vi "PPR_DRIVE_Wheel_ACT.vi"(6 "Pass_Through_Time":dbl=-1.0 format="%33.4f", 9 "Wheel Speed M/S":dbl, 10 "Wheel Speed Dmd M/S":dbl, 11 "Diff Wheel TypDef":T1) -> (3 "Wheel Motor Dmd":dbl, 4 "WheelSpeedErr":dbl, 7 "Limited Speed Dmd M/S":dbl)   [LabVIEW 2019]
uses:
  PPR_DRIVE_Wheel_TYPDEF.ctl
  <vilib>/Rock Robotics/WPI/MotorControl/WPI_MotorControlDeviceRef.ctl
  <vilib>/Rock Robotics/WPI/MotorControl/WPI_MotorControlType.ctl
  <vilib>/Rock Robotics/SystemInterfaces/DIO/FPGA_DIOPWMChannel.ctl
  <vilib>/Rock Robotics/WPI/PWM/WPI_PWMDeadband.ctl
  <vilib>/Rock Robotics/SystemInterfaces/DIO/FPGA_DIOChannel.ctl
  <vilib>/Rock Robotics/WPI/Encoder/WPI_EncoderDevRef.ctl
  <vilib>/Rock Robotics/SystemInterfaces/Encoder/FPGA_EncoderIdx.ctl
  <vilib>/Rock Robotics/SystemInterfaces/Counter/FPGA_CounterCtrSystemIndex.ctl
  <vilib>/Rock Robotics/WPI/Encoder/WPI_EncoderType.ctl
  <vilib>/Rock Robotics/WPI/ThirdParty/JAS_Junk/TrajLib/VI/Util_GetTime_U32.vi
  <vilib>/Rock Robotics/WPI/ThirdParty/JAS_Junk/TrajLib/SlewRateLimiter_New.vi
  <vilib>/Rock Robotics/WPI/ThirdParty/JAS_Junk/TrajLib/SlewRateLimiter_Reset.vi
  <vilib>/Rock Robotics/WPI/ThirdParty/JAS_Junk/TrajLib/SlewRateLimiter_Calculate.vi
  <vilib>/Rock Robotics/WPI/ThirdParty/JAS_Junk/TrajLib/SlewRateLimiter_SetRate.vi
  <vilib>/Rock Robotics/WPI/ThirdParty/JAS_Junk/TrajLib/SimpleMotorFF_Calculate.vi
  <vilib>/Rock Robotics/WPI/ThirdParty/JAS_Junk/TrajLib/PIDController_AtSetpoint.vi
  <vilib>/Rock Robotics/WPI/ThirdParty/JAS_Junk/TrajLib/PIDController_SetPIDF.vi
  <vilib>/Rock Robotics/WPI/ThirdParty/JAS_Junk/TrajLib/PIDController_SetDerivativeFilter.vi
  <vilib>/Rock Robotics/WPI/ThirdParty/JAS_Junk/TrajLib/PIDController_SetIntegratorRange.vi
  <vilib>/Rock Robotics/WPI/ThirdParty/JAS_Junk/TrajLib/PIDController_SetTolerancePandV.vi
  <vilib>/Rock Robotics/WPI/ThirdParty/JAS_Junk/TrajLib/PIDController_DisableContinousInput.vi
  <vilib>/Rock Robotics/WPI/ThirdParty/JAS_Junk/TrajLib/PIDController_EnableContinousInput.vi
  <vilib>/Rock Robotics/WPI/ThirdParty/JAS_Junk/TrajLib/PIDController_Reset.vi
  <vilib>/Rock Robotics/WPI/ThirdParty/JAS_Junk/TrajLib/PIDController_New.vi
  <vilib>/Rock Robotics/WPI/ThirdParty/JAS_Junk/TrajLib/PIDController_SetOutputLimits.vi
  <vilib>/Rock Robotics/WPI/ThirdParty/JAS_Junk/TrajLib/PIDController_NewPeriod.vi
  <vilib>/Rock Robotics/SystemInterfaces/NetworkCommunication/NetComm_UsageReport_report.vi
  <vilib>/Rock Robotics/WPI/ThirdParty/JAS_Junk/TrajLib/VI/Util_GetTime_U64.vi
  PPR_DRIVE_GLOBALS.vi
  <vilib>/Rock Robotics/WPI/ThirdParty/JAS_Junk/TrajLib/Globals/Util_LibraryGlobals.vi
  <vilib>/Rock Robotics/WPI/ThirdParty/JAS_Junk/TrajLib/PIDController_AdvCalculate_FF_Sp_Pv.vi
  <vilib>/Rock Robotics/WPI/ThirdParty/JAS_Junk/TrajLib/Trajectory_Library.lvlib
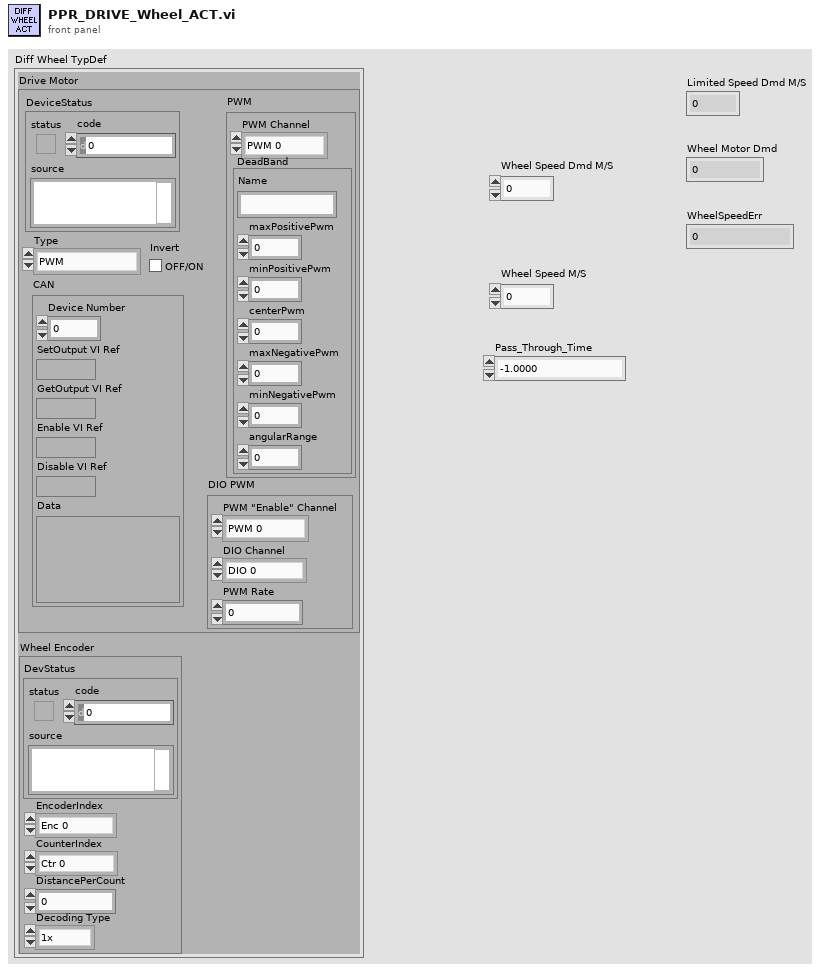
[diagram p1: front panel]
types:
  T1 = typedef "PPR_DRIVE_Wheel_TYPDEF.ctl" = cluster{"Drive Motor":T2, "Wheel Encoder":T7}
  T2 = typedef "WPI_MotorControlDeviceRef.ctl" = cluster{"DeviceStatus":errorcluster, "Type":T3, "PWM":cluster{"PWM Channel":T4, "DeadBand":T5}, "CAN":cluster{"Device Number":u8, "SetOutput VI Ref":variant, "GetOutput VI Ref":variant, "Enable VI Ref":variant, "Disable VI Ref":variant, "Data":variant}, "Invert":bool, "DIO PWM":cluster{"PWM \"Enable\" Channel":T4, "DIOChannel":T6, "PWM Rate":dbl}}
  T3 = typedef "WPI_MotorControlType.ctl" = enum16{"PWM", "CAN", "DIO PWM"}
  T4 = typedef "FPGA_DIOPWMChannel.ctl" = enum8{"PWM 0", "PWM 1", "PWM 2", "PWM 3", "PWM 4", "PWM 5", "PWM 6", "PWM 7", "PWM 8", "PWM 9", "PWM MXP 0", "PWM MXP 1", "PWM MXP 2", "PWM MXP 3", "PWM MXP 4", "PWM MXP 5", "PWM MXP 6", "PWM MXP 7", "PWM MXP 8", "PWM MXP 9", "Invalid"}
  T5 = typedef "WPI_PWMDeadband.ctl" = cluster{"Name":string, "maxPositivePwm":i32, "minPositivePwm":i32, "centerPwm":i32, "maxNegativePwm":i32, "minNegativePwm":i32, "angularRange":u16}
  T6 = typedef "FPGA_DIOChannel.ctl" = enum8{"DIO 0", "DIO 1", "DIO 2", "DIO 3", "DIO 4", "DIO 5", "DIO 6", "DIO 7", "DIO 8", "DIO 9", "DIO MXP 0", "DIO MXP 1", "DIO MXP 2", "DIO MXP 3", "DIO MXP 4", "DIO MXP 5", "DIO MXP 6", "DIO MXP 7", "DIO MXP 8", "DIO MXP 9", "DIO MXP 10", "DIO MXP 11", "DIO MXP 12", "DIO MXP 13", "DIO MXP 14", "DIO MXP 15", "SPI Port CS1", "SPI Port CS2", "SPI Port CS3", "SPI Port MISO", "SPI Port MOSI", "Invalid"}
  T7 = typedef "WPI_EncoderDevRef.ctl" = cluster{"DevStatus":errorcluster, "EncoderIndex":T8, "CounterIndex":T9, "DistancePerCount":dbl, "Decoding Type":T10}
  T8 = typedef "FPGA_EncoderIdx.ctl" = enum8{"Enc 0", "Enc 1", "Enc 2", "Enc 3", "Enc 4", "Enc 5", "Enc 6", "Enc 7", "Invalid"}
  T9 = typedef "FPGA_CounterCtrSystemIndex.ctl" = enum8{"Ctr 0", "Ctr 1", "Ctr 2", "Ctr 3", "Ctr 4", "Ctr 5", "Ctr 6", "Ctr 7", "Invalid"}
  T10 = typedef "WPI_EncoderType.ctl" = enum16{"1x", "2x", "4x"}
  T11 = typedef "Trajectory_Library.lvlib/SIMPLE_MOTOR_FF.ctl" = cluster{"Ks":dbl, "Kv":dbl, "Ka":dbl, "KnInv":dbl}
  T12 = typedef "Trajectory_Library.lvlib/PID_ADV_LIMITS.ctl" = cluster{"MaxInput":dbl, "MinInput":dbl, "Continuous":bool, "MaxOutput":dbl, "MinOutput":dbl}
  T13 = typedef "Trajectory_Library.lvlib/PID_ADV_TUNING.ctl" = cluster{"Kf":dbl, "Kp":dbl, "Ki":dbl, "Kd":dbl, "MaximumIntegral":dbl, "MinimumIntegral":dbl, "Filter Derivative":bool}
  T14 = typedef "Trajectory_Library.lvlib/PID_CONTROLLER.ctl" = cluster{"Kp":dbl, "Ki":dbl, "Kd":dbl, "Period":dbl, "Max_Integral":dbl, "Min_Integral":dbl, "Max_Input":dbl, "Min_Input":dbl, "Continuous":bool, "PositionError":dbl, "VelocityError":dbl, "PrevError":dbl, "TotalError":dbl, "PositionTolerance":dbl, "VelocityTolerance":dbl, "SetPoint":dbl, "Kf":dbl, "Prev_Deriv":dbl, "Prev_Deriv 2":dbl, "DerivativeFilter":bool, "Min_Output":dbl, "Max_Output":dbl, "Prev_F_P":dbl, "Prev_F_P_2":dbl, "AntiWindupActive":bool, "Measurement":dbl}
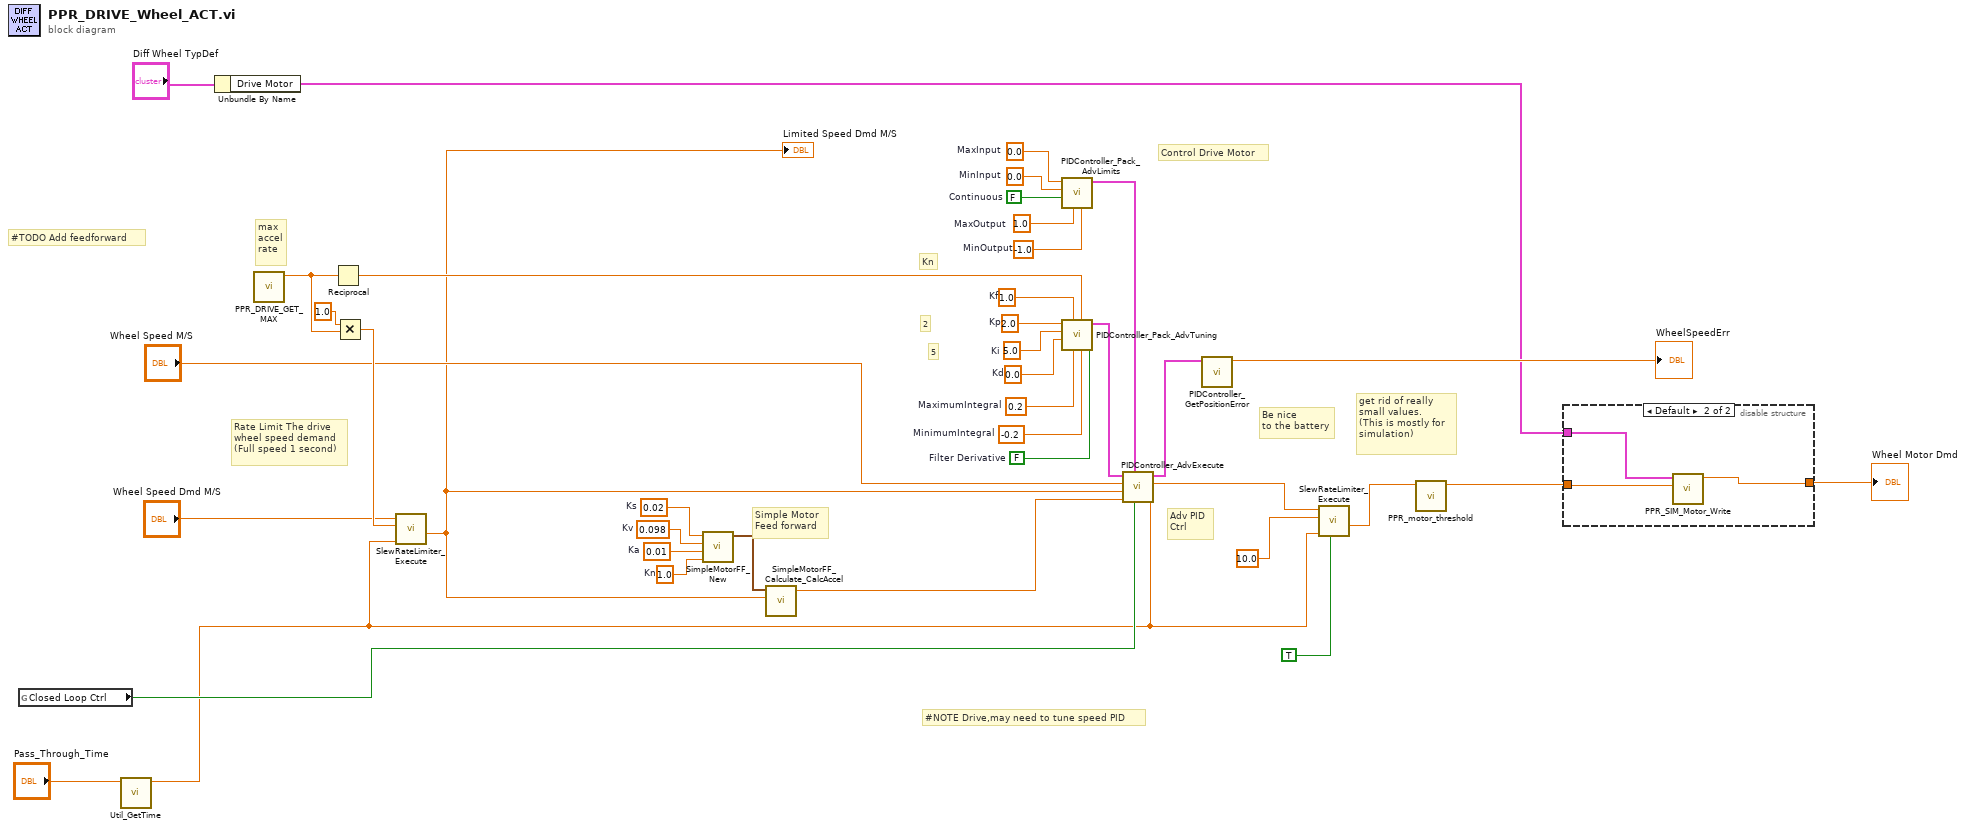
[diagram p0: block diagram]
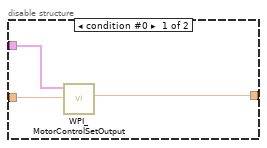
[diagram p2: hidden frame]
diagram:
  w7 = 1.0  # Kn
  w5 = 0.02  # Ks
  w4 = 0.098  # Kv
  w3 = 0.01  # Ka
  w35 = 2.0  # Kp
  w34 = 5.0  # Ki
  w33 = 0.0  # Kd
  w32 = 1.0  # Kf
  w31 = 0.2  # MaximumIntegral
  w30 = -0.2  # MinimumIntegral
  w29 = FALSE  # Filter Derivative
  w27 = 0.0  # MinInput
  w26 = FALSE  # Continuous
  w25 = 1.0  # MaxOutput
  w28 = -1.0  # MinOutput
  w24 = 0.0  # MaxInput
  # "Simple Motor\nFeed forward"
  # "#TODO Add feedforward"
  # "Control Drive Motor"
  # "Be nice\nto the battery"
  # "5"
  # "2"
  # "Kn"
  # "Adv PID\nCtrl"
  # "Rate Limit The drive\nwheel speed demand\n(Full speed 1 second)"
  # "#NOTE Drive,may need to tune speed PID"
  # "get rid of really\nsmall values.\n(This is mostly for \nsimulation)"
  # "max\naccel\nrate"
  n1 = global read "PPR_DRIVE_GLOBALS.vi" "Closed Loop Ctrl"() -> (w11:bool)
  n2 = call <vilib>:"Util_GetTime.vi"("Pass_Through_Time"="Pass_Through_Time") -> ("FPGA_Time_Seconds"=w10:dbl)  [unwired: 8 in, 2 out]
  n3 = Unbundle By Name("Diff Wheel TypDef") -> ("Drive Motor"=w18:T2)
  n4 = call "PPR_DRIVE_GET_MAX.vi"() -> ("Max Wheel Vel (Meter/Sec)"=w38:dbl)  [unwired: 10 in, 1 out]
  n5 = Reciprocal(x=w38) -> (1/x=w21:dbl)
  n6 = Multiply(x=1.0, y=w38) -> (x*y=w37:dbl)
  n7 = call <vilib>:"SlewRateLimiter_Execute.vi"("Time"=w10, "PositiveRate"=w37, "Input"="Wheel Speed Dmd M/S") -> ("Output"=w2:dbl)  [unwired: 7 in, 1 out]
  "Limited Speed Dmd M/S" <- w2
  n8 = call <vilib>:"SimpleMotorFF_New.vi"("Kn"=w7, "Ka"=w3, "Kv"=w4, "Ks"=w5) -> ("SIMPLE_MOTOR_FF"=w6:T11)  [unwired: 7 in]
  n9 = call <vilib>:"SimpleMotorFF_Calculate_CalcAccel.vi"("VelSp"=w2, "SIMPLE_MOTOR_FF"=w6) -> ("FeedForward"=w1:dbl)  [unwired: 9 in]
  n10 = call <vilib>:"PIDController_Pack_AdvLimits.vi"("MinOutput"=w28, "MaxOutput"=w25, "Continuous"=w26, "MinInput"=w27, "MaxInput"=w24) -> ("Adv PID Limits"=w22:T12)  [unwired: 6 in]
  n11 = call <vilib>:"PIDController_Pack_AdvTuning.vi"("Filter Derivative"=w29, "MinimumIntegral"=w30, "Kn"=w21, "MaximumIntegral"=w31, "Kf"=w32, "Kd"=w33, "Ki"=w34, "Kp"=w35) -> ("Adv PID Tuning"=w23:T13)  [unwired: 3 in]
  n12 = call <vilib>:"PIDController_AdvExecute.vi"("Time"=w10, "Auto"=w11, "Adv PID Limits"=w22, "FF-FeedForward"=w1, "SP-SetPoint"=w2, "PV-Measurement"="Wheel Speed M/S", "Adv PID Tuning"=w23) -> ("CO-ControlOutput"=w15:dbl, "out PID_CONTROLLER"=w20:T14)  [unwired: 2 in, 1 out]
  n13 = call <vilib>:"PIDController_GetPositionError.vi"("in PID_CONTROLLER"=w20) -> ("PositionError"=→"WheelSpeedErr":dbl)  [unwired: 10 in]
  n14 = call <vilib>:"SlewRateLimiter_Execute.vi"("Enable"=TRUE, "Time"=w10, "PositiveRate"=10.0, "Input"=w15) -> ("Output"=w14:dbl)  [unwired: 6 in, 1 out]
  n15 = call "PPR_motor_threshold.vi"("motor in"=w14) -> ("motor out"=w17:dbl)  [unwired: 10 in]
  n16 = disable-structure shown="Default" {
    disable-tunnel: w17 -> [w43 w45]
    disable-tunnel: w18 -> [w42 w46]
    disable-tunnel: [w41 w44] -> w16
    frame condition #0 {
      n17 = call <vilib>:"WPI_MotorControlSetOutput.vi"("Output"=w43, "MotorControlDevRef"=w42) -> ("Motor Output"=w41:dbl)  [unwired: 7 in, 2 out]
    }
    frame condition #1 (active) {
      n18 = call "PPR_SIM_Motor_Write.vi"("Motor Demand"=w45, "Motor Device Reference"=w46) -> ("Out Motor Demand"=w44:dbl)  [unwired: 9 in]
    }
  }
  "Wheel Motor Dmd" <- w16
